vi "FRCts20_Backend_ObtainReturnSpecific.vi"(8 "error in (no error)":errorcluster, 10 "Elements to search":i32, 11 "Key in":string) -> (0 "error out":errorcluster, 3 "Message Value":string)   [LabVIEW 2013, in "FRCts20_Backend_Engine.lvlib"]
doc: "Searches through the AMC queue for a specific key, once we know the key exists. Non reentrant to prevent race conditions between accessing processes."
uses:
  FRCts20_Backend_Engine.lvlib
  FRCts20_Backend_DequeueDataOperations.ctl
  FRCts20_Backend_FGVOperation.ctl
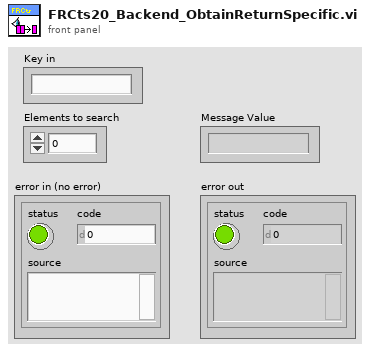
[diagram p1: front panel]
types:
  T1 = typedef "FRCts20_Backend_Engine.lvlib/FRCts20_Backend_DequeueDataOperations.ctl" = enum16{"Initialize", "DequeueDataReturn", "GetQueues"}
  T2 = typedef "FRCts20_Backend_Engine.lvlib/FRCts20_Backend_FGVOperation.ctl" = enum16{"Initialize", "EnqueueMessage", "EnqueueDataReturn", "FlushMessage", "FlushDataReturn"}
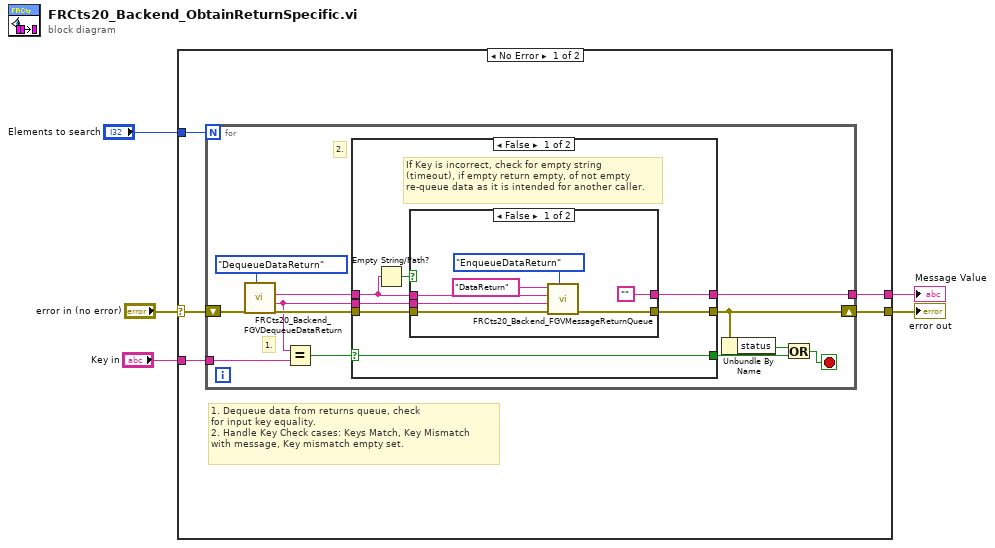
[diagram p0: block diagram]
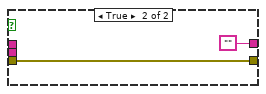
[diagram p2: hidden frame]
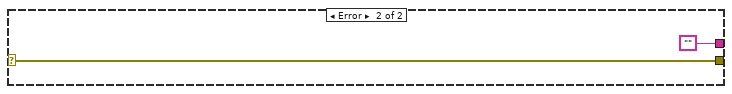
[diagram p4: hidden frame]
diagram:
  n1 = case shown="No Error" "error in (no error)" {
    selector: "error in (no error)" -> [w10 w43]
    tunnel: [w9 w43] -> w2
    tunnel: "Key in" -> [w8 _]
    tunnel: [w7 ""] -> w3
    tunnel: "Elements to search" -> [w6 _]
    frame No Error {
      # "1. Dequeue data from returns queue, check\nfor input key equality.\n2. Handle Key Check cases: Keys Match, Key Mismatch\nwith message, Key mismatch empty set."
      n2 = for {
        N: w6 -> [_]
        shift-right: [w17] -> w9
        shift-left: w10 -> [w22]
        tunnel: w8 -> [w20]
        tunnel: [w12] -> w7
        stop <- w11 stop-if-true
        # "2."
        # "1."
        n3 = call "FRCts20_Backend_FGVDequeueDataReturn.vi"("Operation"=FRCts20_Backend_DequeueDataOperations."DequeueDataReturn", "error in (no error)"=w22) -> ("error out"=w18:errorcluster, "Key"=w13:string, "Message Value"=w14:string)  [unwired: 5 in, 2 out]
        n4 = Equal?(x=w13, y=w20) -> (x = y?=w19:bool)
        n5 = case shown="False" w19 {
          selector: w19 -> [w24 w40]
          tunnel: w18 -> [w28 w41]
          tunnel: [w27 w41] -> w17
          tunnel: [w24 w40] -> w15
          tunnel: w14 -> [w25 w39]
          tunnel: [w26 w39] -> w12
          tunnel: w13 -> [w23 _]
          frame False {
            # "If Key is incorrect, check for empty string \n(timeout), if empty return empty, of not empty\nre-queue data as it is intended for another caller."
            n6 = Empty String/Path?(string/path=w25) -> (empty?=w29:bool)
            n7 = case shown="False" w29 {
              tunnel: w28 -> [w36 w38]
              tunnel: [w35 w38] -> w27
              tunnel: ["" ""] -> w26
              tunnel: w25 -> [w33 _]
              tunnel: w23 -> [w30 _]
              frame False {
                n8 = call "FRCts20_Backend_FGVMessageReturnQueue.vi"("Operation"=FRCts20_Backend_FGVOperation."EnqueueDataReturn", "error in (no error)"=w36, "Key"=w30, "Message Value"=w33, "Message Name"="DataReturn") -> ("error out"=w35:errorcluster)  [unwired: 5 in, 1 out]
              }
              frame True {
              }
            }
          }
          frame True {
            # "If Key is correct, return Message Value\nto the caller."
          }
        }
        n9 = Unbundle By Name(w17) -> ("status"=w16:bool)
        n10 = Or(x=w16, y=w15) -> (x .or. y?=w11:bool)
      }
    }
    frame Error {
    }
  }
  "Message Value" <- w3
  "error out" <- w2
